vi "Stop.vi"(8 "error in (no error)":errorcluster, 11 "ArrayManager in":refnum<class "ArrayManager.lvclass">) -> (0 "error out":errorcluster, 3 "ArrayManager out":refnum<class "ArrayManager.lvclass">)   [LabVIEW 2020, in "OOPanel.lvlib" / "ArrayManager.lvclass"]
uses:
  ArrayManager.lvclass
  ArrayManager.lvclass/ArrayManager.ctl
panel:
  out "call chain":string[](array[string])
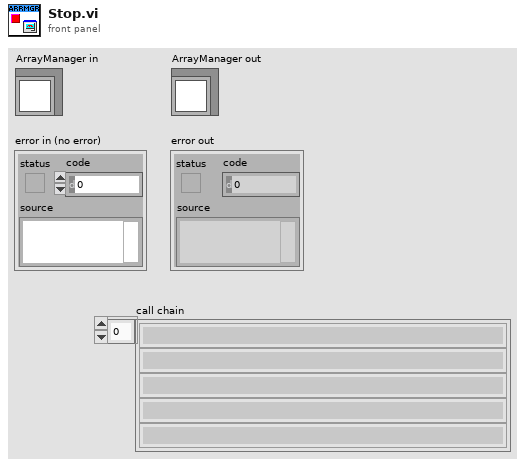
[diagram p1: front panel]
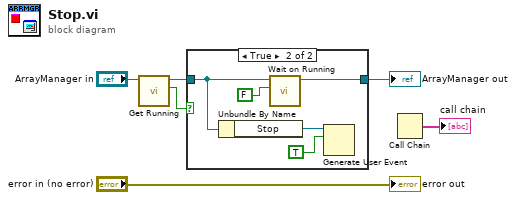
[diagram p0: block diagram]
diagram:
  n1 = call "Get Running.vi"("ArrayManager in"="ArrayManager in") -> ("Running"=w2:bool, "ArrayManager out"=w4:refnum<class "ArrayManager.lvclass">)  [unwired: 8 in, 1 out]
  n2 = case shown="True" w2 {
    tunnel: w4 -> [w7 w10]
    tunnel: [w7 w9] -> w3
    frame False {
    }
    frame True {
      n3 = Unbundle By Name(w10) -> ("Stop"=w12:refnum<user-event>)
      n4 = call "Wait on Running.vi"("Value"=FALSE, "ArrayManager in"=w10) -> ("ArrayManager out"=w9:refnum<class "ArrayManager.lvclass">)  [unwired: 8 in, 1 out]
      n5 = Generate User Event(user event=w12, event data cluster=TRUE ("event data")) -> ()  [unwired: 2 in, 2 out]
    }
  }
  "ArrayManager out" <- w3
  n6 = Call Chain() -> (call chain=→"call chain":string[])
  "error out" <- "error in (no error)"
